vi "Global - All RT Loop Stop.vi"() -> ()   [LabVIEW 2022 SP3]
panel:
  in  "All RT Loop Stop":bool
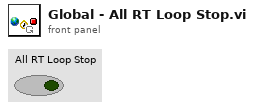
[diagram p1: front panel]
diagram:
